vi "MapCreator.vi"(0 "reference in":refnum<class "Map.lvclass">, 1 "Path":path, 5 "error in (no error)":errorcluster) -> (14 "reference out":refnum<class "Map.lvclass">, 19 "error out":errorcluster)   [LabVIEW 2019, in "Map.lvclass"]
doc: "This VI creates the Map"
uses:
  Map.lvclass
  <vilib>/picture/picture.llb/imagedata.ctl
panel:
  out "Array":bool[][](array[boolean])
  out "Picture":picture
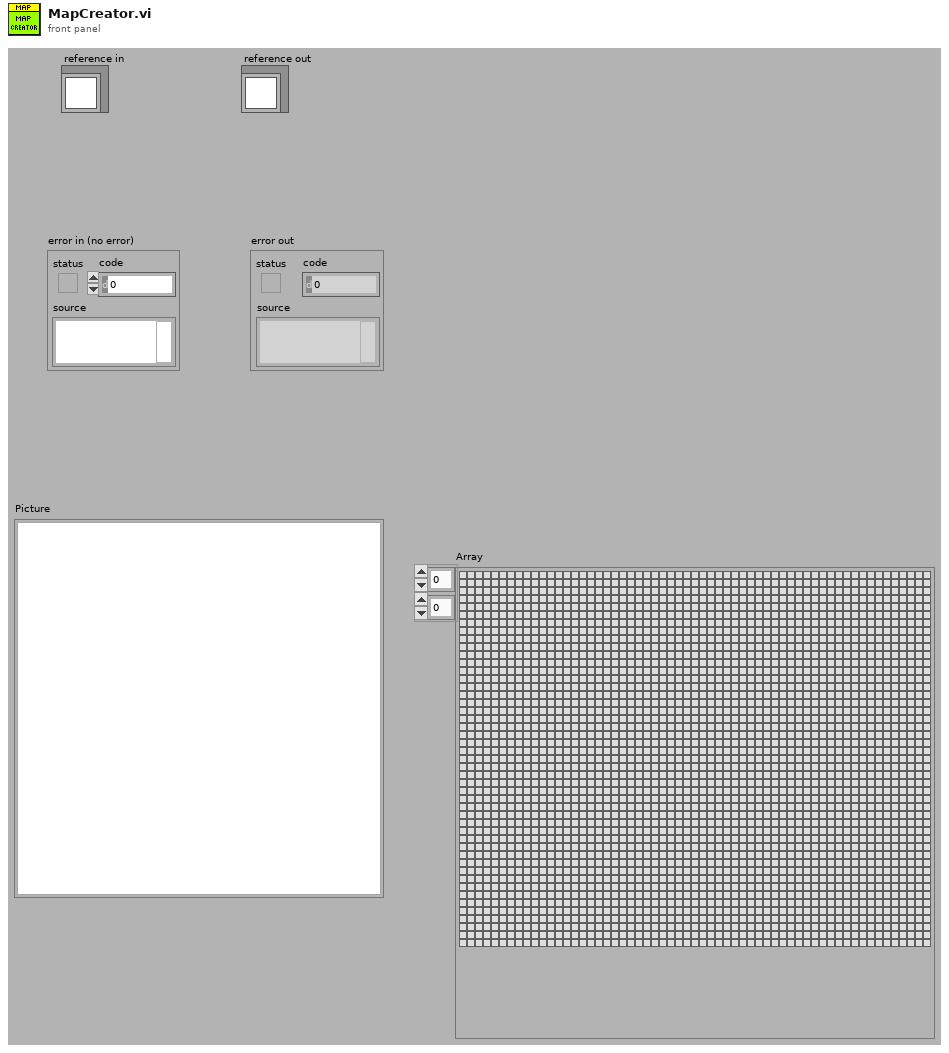
[diagram p1: front panel]
types:
  T1 = typedef "imagedata.ctl" = cluster{"image type":i32, "image depth":i32, "image":u8[], "mask":u8[], "colors":u32[], "Rectangle":cluster{"left":i16, "top":i16, "right":i16, "bottom":i16}}
  T2 = typedef "Map.lvclass/ObjectAttributes.ctl" = cluster{"Width":i32, "Height":i32, "Map":bool[][]}
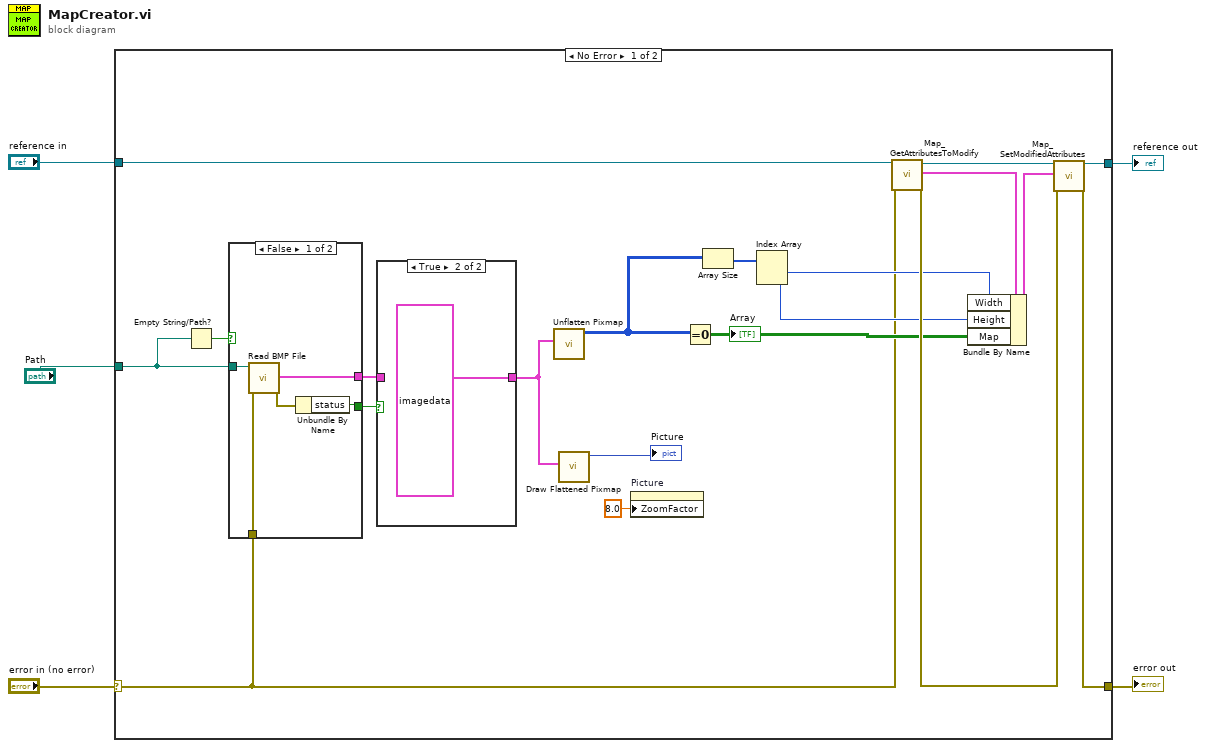
[diagram p0: block diagram]
diagram:
  n1 = case shown="No Error" "error in (no error)" {
    selector: "error in (no error)" -> [w8 w35]
    tunnel: [w24 w35] -> w4
    tunnel: [w22 w34] -> w2
    tunnel: "reference in" -> [w23 w34]
    tunnel: "Path" -> [w7 _]
    frame No Error {
      n2 = Empty String/Path?(string/path=w7) -> (empty?=w6:bool)
      n3 = case shown="False" w6 {
        selector: w6 -> [_ w31]
        tunnel: w8 -> [w30 _]
        tunnel: [w29 _] -> w10
        tunnel: w7 -> [w28 _]
        tunnel: [w26 w31] -> w9
        frame False {
          n4 = call <vilib>:"Read BMP File.vi"("error in (no error)"=w30, "path to BMP file"=w28) -> ("error out"=w27:errorcluster, "image data"=w29:T1)  [unwired: 8 out]
          n5 = Unbundle By Name(w27) -> ("status"=w26:bool)
        }
        frame True {
        }
      }
      n6 = case shown="True" w9 {
        tunnel: w10 -> [w32 _]
        tunnel: [w32 T1 {"image type"=0, "image depth"=24, "image"=array[6210 elements], "mask"=[], "colors"=[], "Rectangle"={"left"=0, "top"=0, "right"=45, "bottom"=46}} ("image data")] -> w13
        frame False {
        }
        frame True {
        }
      }
      n7 = call <vilib>:"Unflatten Pixmap.vi"("image data"=w13) -> ("24-bit pixmap"=w17:u32[][])  [unwired: 10 out]
      n8 = call <vilib>:"Draw Flattened Pixmap.vi"("image data"=w13) -> ("new picture"=→"Picture":picture)  [unwired: 1 in, 7 out]
      n9 = property on="Picture" class="Pict"("ZoomFactor"=sgl 8.0 ("Zoom Factor")) -> ()  [unwired: 2 in, 2 out]
      n10 = Equal To 0?(x=w17) -> (x = 0?=w19:bool[][])
      "Array" <- w19
      n11 = Array Size(array=w17) -> (size(s)=w16:i32[])
      n12 = Index Array(array=w16) -> (element #1=w15:i32, element #2=w14:i32)  [unwired: 2 in]
      n13 = call "Map_GetAttributesToModify.vi"("reference in"=w23, "error in (no error)"=w8) -> ("reference out"=w25:refnum<class "Map.lvclass">, "Attributes"=w12:T2, "error out"=w21:errorcluster)  [unwired: 1 in, 14 out]
      n14 = Bundle By Name(cluster=w12, "Width"=w15, "Height"=w14, "Map"=w19) -> (w11:T2)
      n15 = call "Map_SetModifiedAttributes.vi"("reference in"=w25, "Attributes"=w11, "error in (no error)"=w21) -> ("reference out"=w22:refnum<class "Map.lvclass">, "error out"=w24:errorcluster)  [unwired: 3 in, 12 out]
    }
    frame Error {
    }
  }
  "error out" <- w4
  "reference out" <- w2
